vi "Get Server Internal UEs.vi"(11 "OOP Server in":refnum<class "Temperature_server.lvclass">) -> (2 "Server Internal UEs":T1, 3 "OOP Server out":refnum<class "Temperature_server.lvclass">)   [LabVIEW 2019, in "Temperature_server.lvlib" / "Temperature_server.lvclass"]
uses:
  Temperature_server.lvclass
  typeDefs/Server Internal UEs.ctl
  typeDefs/Server Internal Message.ctl
  Temperature_server.lvclass/Temperature_server.ctl
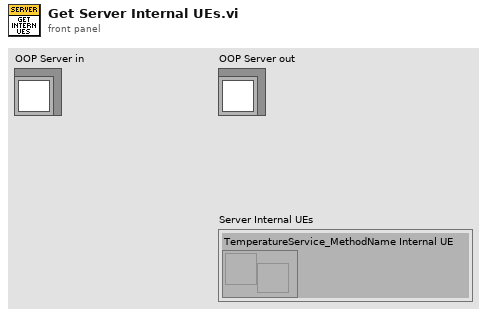
[diagram p1: front panel]
types:
  T1 = typedef "Temperature_server.lvlib/Temperature_server.lvclass/Server Internal UEs.ctl" = cluster{"TemperatureService_MethodName Internal UE":refnum<user-event>}
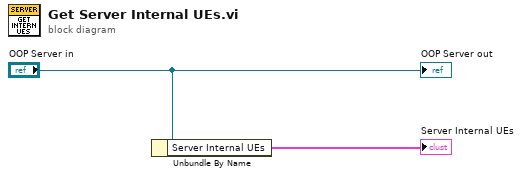
[diagram p0: block diagram]
diagram:
  n1 = Unbundle By Name("OOP Server in") -> ("Server Internal UEs"=→"Server Internal UEs":T1)
  "OOP Server out" <- "OOP Server in"
